vi "ir test.vi"() -> ()   [LabVIEW 2012, in "Testing.lvrbt"]
uses:
  Testing.lvrbt
  <vilib>/NXT/Dual Mode Library/Waits/Wait_Num(msec).vi
  <vilib>/NXT/LegoClasses/BrickReference/BrickReference.lvclass
  <vilib>/NXT/Subs/LVHSConnector.ctl
  <vilib>/NXT/NXTIO Xnodes/NXTIOXNode/NXTIO.xnode
  <vilib>/NXT/Hardware/Plugins/Open Port/OpenPortAddress.ctl
  <vilib>/NXT/NXTIO Xnodes/AddressXNode/NXTIOAddress.xnode
panel:
  out "Enabled":bool
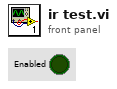
[diagram p1: front panel]
types:
  T1 = typedef "OpenPortAddress.ctl" = i32
  T2 = typedef "LVHSConnector.ctl" = refnum<class "BrickReference.lvclass">
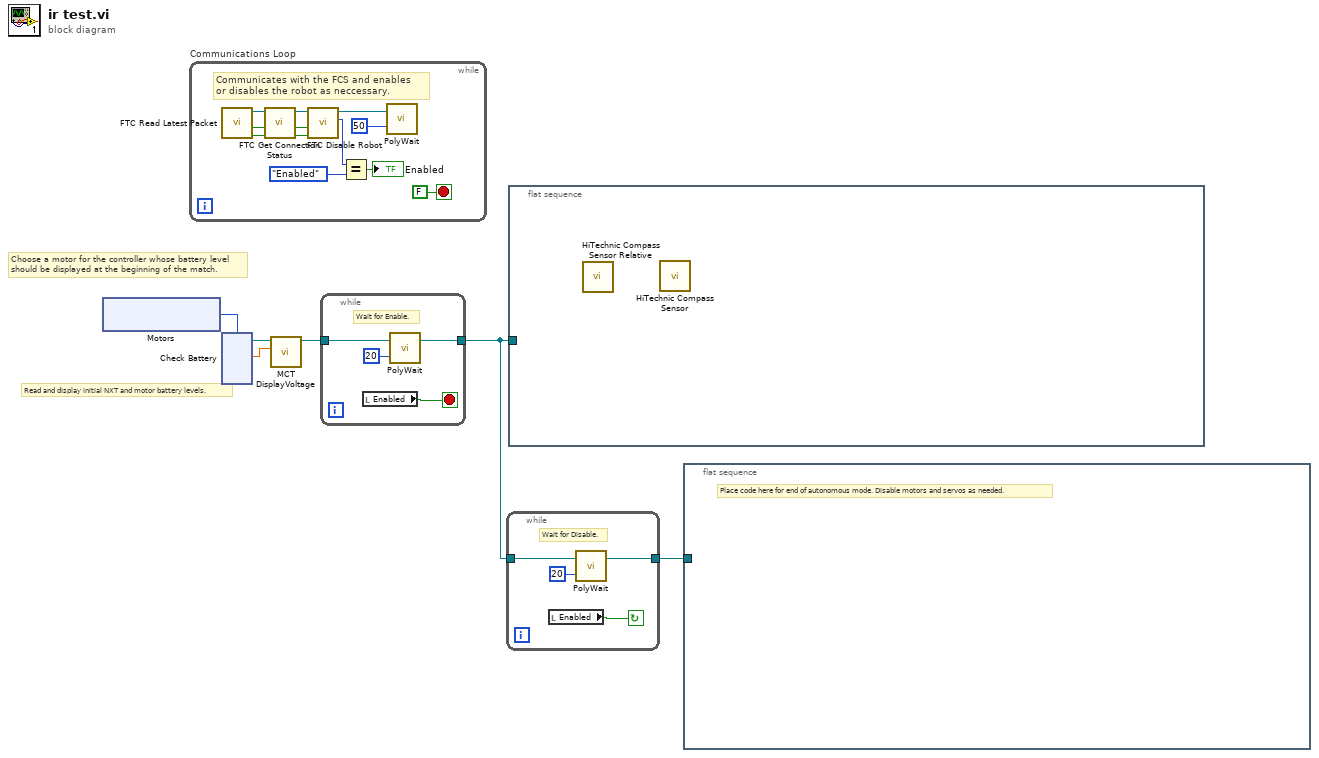
[diagram p0: block diagram]
diagram:
  # "Read and display initial NXT and motor battery levels."
  # "Choose a motor for the controller whose battery level \nshould be displayed at the beginning of the match."
  n1 = xnode "Motors"() -> ("Motor"=w1:T1)
  n2 = while "Communications Loop" {
    stop <- FALSE stop-if-true
    # "Communicates with the FCS and enables \nor disables the robot as neccessary."
    n3 = call <vilib>:"FTC Read Latest Packet.vi"() -> ("Packet Received?"=w16:bool, "Stopped?"=w15:bool, "NXT/EV3"=w18:T2)  [unwired: 6 in, 3 out]
    n4 = call <vilib>:"FTC Get Connection Status.vi"("Packet Received?"=w16, "Stopped?"=w15, "NXT/EV3"=w18) -> ("Online?"=w7:bool, "Stopped?"=w8:bool, "NXT/EV3"=w17:T2)  [unwired: 5 in]
    n5 = call <vilib>:"FTC Disable Robot.vi"("Online?"=w7, "Stopped?"=w8, "NXT/EV3"=w17) -> ("Enabled?"=w11:enum16{"Disabled", "Enabled"}, "NXT/EV3"=w13:T2)  [unwired: 3 in]
    n6 = Equal?(x=w11, y=enum16{"Disabled", "Enabled"}."Enabled") -> (x = y?=→"Enabled":bool)
    n7 = call-poly <vilib>:"PolyWait.vi"("Time (100 msec)"=u32 50 ("Time (msec)"), "NXT/EV3"=w13) -> ()  [unwired: 2 in, 1 out]
  }
  n8 = xnode "Check Battery"("Motors"=w1) -> ("Voltage 1"=w2:sgl, "NXT/EV3"=w4:T2)  [unwired: 1 in]
  n9 = call <vilib>:"MCT DisplayVoltage.vi"("Motor Voltage"=w2, "NXT/EV3"=w4) -> ("NXT/EV3"=w3:T2)  [unwired: 9 in]
  n10 = while {
    tunnel: [w20] -> w6
    tunnel: w3 -> [w19]
    stop <- w21 stop-if-true
    # "Wait for Enable."
    n11 = local read "Enabled"() -> (w21:bool)
    n12 = call-poly <vilib>:"PolyWait.vi"("Time (100 msec)"=u32 20 ("Time (msec)"), "NXT/EV3"=w19) -> ("NXT/EV3"=w20:T2)  [unwired: 2 in]
  }
  n13 = while {
    tunnel: [w24] -> w5
    tunnel: w6 -> [w23]
    stop <- w25 continue-if-true
    # "Wait for Disable."
    n14 = local read "Enabled"() -> (w25:bool)
    n15 = call-poly <vilib>:"PolyWait.vi"("Time (100 msec)"=u32 20 ("Time (msec)"), "NXT/EV3"=w23) -> ("NXT/EV3"=w24:T2)  [unwired: 2 in]
  }
  n16 = flat-sequence {
    tunnel: w6 -> [_]
    frame #0 {
      n17 = call <vilib>:"HiTechnic Compass Sensor Relative.vi"() -> ()  [unwired: 3 in, 2 out]
      n18 = call <vilib>:"HiTechnic Compass Sensor.vi"() -> ()  [unwired: 3 in, 2 out]
    }
  }
  n19 = flat-sequence {
    tunnel: w5 -> [_]
    frame #0 {
      # "Place code here for end of autonomous mode. Disable motors and servos as needed."
    }
  }
